vi "Process var.vi"() -> ()   [LabVIEW 2016]
panel:
  out "多参数输出":T1 {"浊度"."mean" format="%0.2f"; "电导率"."mean" format="%0.2f"; "DO"."mean" format="%0.2f"; "pH"."mean" format="%0.2f"; "水温"."mean" format="%0.2f"}
  out "CODcr参数输出":T2 {"跨度参数输出"."mean" format="%0.2f"; "零点参数输出"."mean" format="%0.2f"; "水样参数输出"."mean" format="%0.2f"}
  out "CODMn参数输出":T2 {"跨度参数输出"."mean" format="%0.2f"; "零点参数输出"."mean" format="%0.2f"; "水样参数输出"."mean" format="%0.2f"}
  out "TN参数输出":T2 {"跨度参数输出"."mean" format="%0.2f"; "零点参数输出"."mean" format="%0.2f"; "水样参数输出"."mean" format="%0.2f"}
  out "TP参数输出":T2 {"跨度参数输出"."mean" format="%0.2f"; "零点参数输出"."mean" format="%0.2f"; "水样参数输出"."mean" format="%0.2f"}
  out "NH3N参数输出":T2 {"跨度参数输出"."mean" format="%0.2f"; "零点参数输出"."mean" format="%0.2f"; "水样参数输出"."mean" format="%0.2f"}
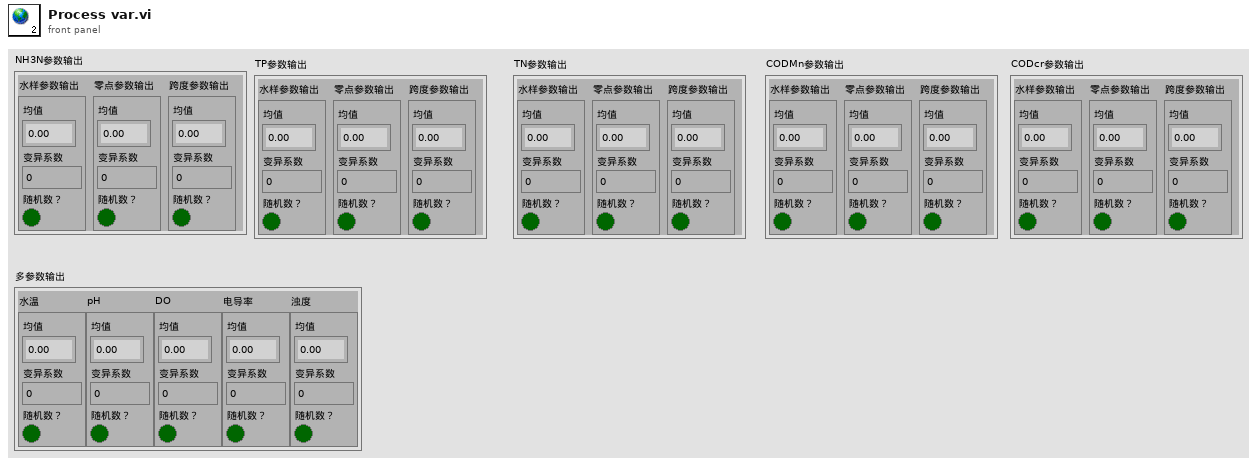
[diagram p1: front panel]
types:
  T1 = cluster{"水温":cluster{"mean":dbl, "变异系数":dbl, "随机数？":bool}, "pH":cluster{"mean":dbl, "变异系数":dbl, "随机数？":bool}, "DO":cluster{"mean":dbl, "变异系数":dbl, "随机数？":bool}, "电导率":cluster{"mean":dbl, "变异系数":dbl, "随机数？":bool}, "浊度":cluster{"mean":dbl, "变异系数":dbl, "随机数？":bool}}
  T2 = cluster{"水样参数输出":cluster{"mean":dbl, "变异系数":dbl, "随机数？":bool}, "零点参数输出":cluster{"mean":dbl, "变异系数":dbl, "随机数？":bool}, "跨度参数输出":cluster{"mean":dbl, "变异系数":dbl, "随机数？":bool}}
diagram:
